vi "control command.vi"(8 "error in (no error)":errorcluster, 9 "data":u16, 10 "axis":u16, 11 "head":u16) -> (0 "error out":errorcluster)   [LabVIEW 2015, in "SCANalone4x64.lvlib"]
doc: "__declspec(dllimport) void __stdcall control_command(unsigned short head, unsigned short axis, unsigned short data);"
uses:
  <userlib>/SCANalone4x64/SCANalone4x64.lvlib
  <userlib>/SCANalone4x64/SCANalone4x64.dll
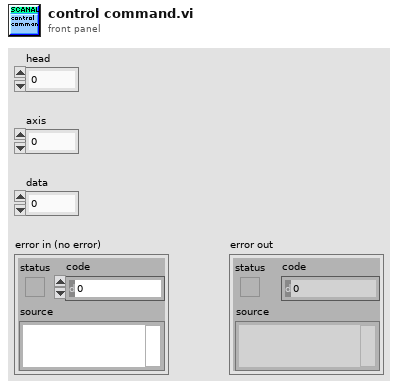
[diagram p1: front panel]
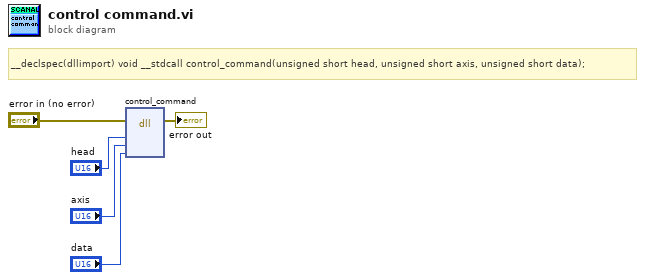
[diagram p0: block diagram]
diagram:
  # "__declspec(dllimport) void __stdcall control_command(unsigned short head, unsigned short axis, unsigned short data);"
  n1 = dll-call lib="C:/Program Files/National Instruments/LabVIEW 2015/user.lib/SCANalone4x64/SCANalone4x64.*" fn="control_command"(error in="error in (no error)", "head"="head", "axis"="axis", "data"="data") -> (error out=→"error out":errorcluster)  [unwired: 6 in, 1 out]
